vi "lv_mutipleTable.vi"(6 "buf_len":i32) -> (5 "out_table":i32[](array[numeric]), 7 "status":i32)   [LabVIEW 2026]
uses:
  vision_core_c/bin/math_formulas.dll
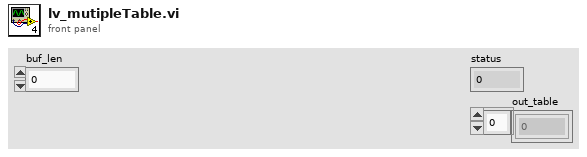
[diagram p1: front panel]
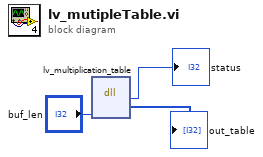
[diagram p0: block diagram]
diagram:
  n1 = dll-call lib="D:/git_proj/LabC-Vision/vision_core_c/bin/math_formulas.dll" fn="lv_multiplication_table"("buf_len"="buf_len") -> ("return type"=→"status":i32, "out_table"=→"out_table":i32[])  [unwired: 5 in, 2 out]
